vi "main.eng.proc-insert-instructions.vi"(8 "error in (no error)":errorcluster, 9 "instructions in":variant[](array[variant]), 10 "procedureName":string, 11 "procs in":cluster{"Procedure":variant[]}[](array[cluster])) -> (0 "error out":errorcluster, 3 "procs out":cluster{"Procedure":variant[]}[](array[cluster]))   [LabVIEW 2024]
uses:
  controls/typeProcVarientName.ctl
  Polymorphics/variantCtrlNumber.vi
  proc.util.validateParamExist.vi
  <vilib>/Utility/error.llb/Clear Errors.vi
  util.error.create.vi
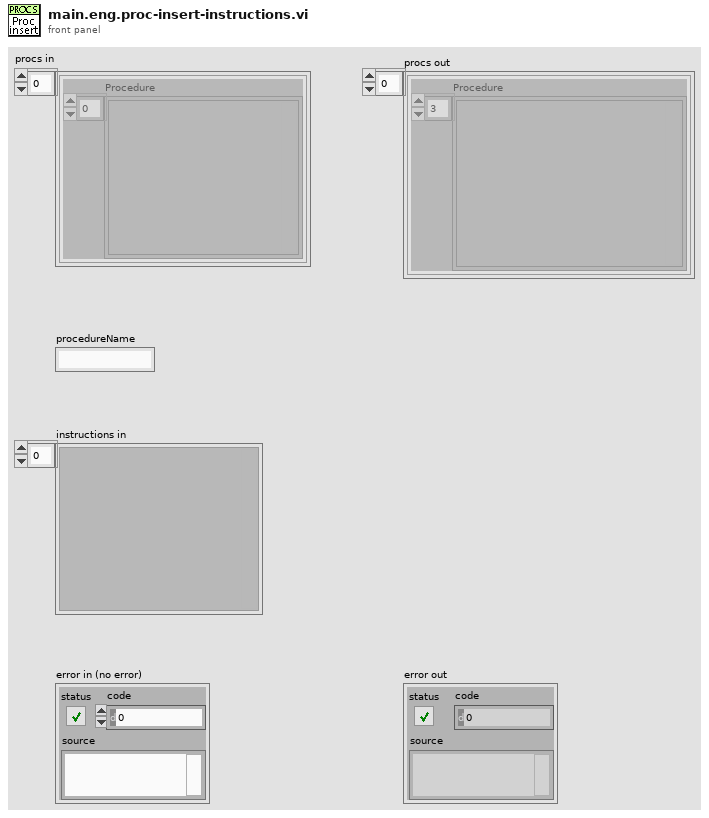
[diagram p1: front panel]
types:
  T1 = typedef "typeProcVarientName.ctl" = enum16{"procNameID", "procModuleID", "procPath", "procIsRunning", "procIndex", "procModule", "procRegisterNumeric", "procRegisterString", "procReport", "procReportPrev", "procCLK", "procStepPointer", "procType"}
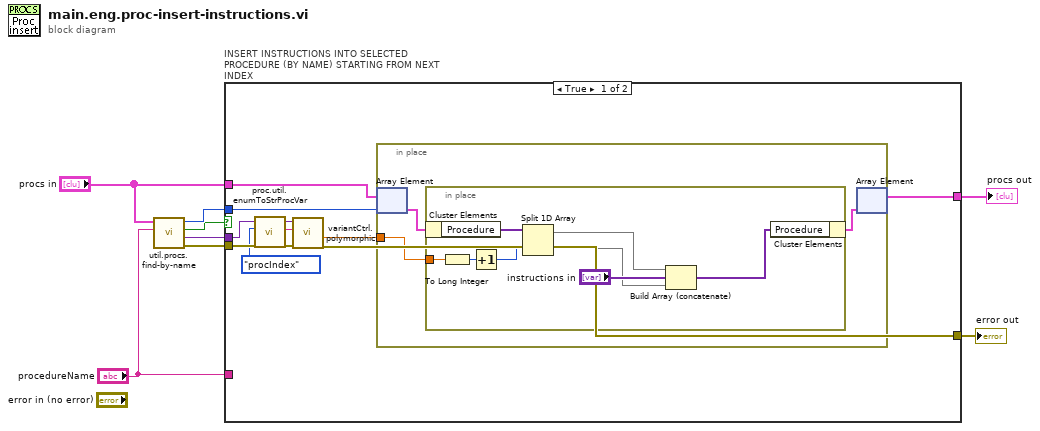
[diagram p0: block diagram]
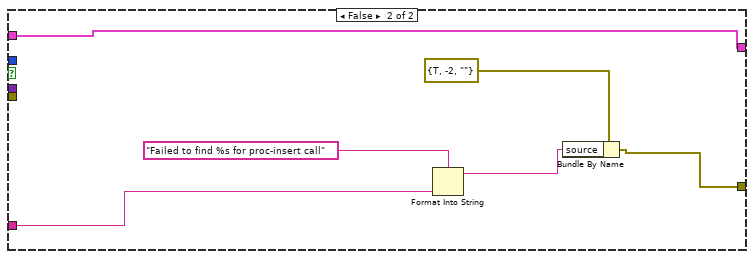
[diagram p2: hidden frame]
diagram:
  n1 = call "util.procs.find-by-name.vi"("ProcName in"="procedureName", "Procs in"="procs in") -> ("error out"=w3:errorcluster, "ProcHead"=w2:variant, "Found?"=w1:bool, "procIndex"=w5:i32)  [unwired: 4 in, 2 out]
  n2 = case "INSERT INSTRUCTIONS INTO SELECTED PROCEDURE (BY NAME) STARTING FROM NEXT INDEX" shown="True" w1 {
    tunnel: [w17 w34] -> w8
    tunnel: "procedureName" -> [_ w33]
    tunnel: "procs in" -> [w16 w32]
    tunnel: w5 -> [w15 _]
    tunnel: [w14 w32] -> w4
    tunnel: w3 -> [w13 _]
    tunnel: w2 -> [w12 _]
    frame True {
      n3 = call "proc.util.enumToStrProcVar.vi"("Proc var"=typeProcVarientName."procIndex" ("name")) -> ("String"=w10:string)  [unwired: 10 in]
      n4 = call-poly "variantCtrl.polymorphic.vi"("error in"=w13, "name in"=w10, "variant in"=w12) -> ("error out"=w17:errorcluster, "number"=w11:dbl)  [unwired: 5 in, 2 out]
      n5 = in-place {
        in-place-border: w11 -> [w20]
        n6 = in-place-array #1(w16, w15) -> (w19:cluster{"Procedure":variant[]})
        n7 = in-place {
          in-place-border: w20 -> [w28]
          n8 = in-place-cluster #2(w19) -> ("Procedure"=w26:variant[])
          n9 = To Long Integer(number=w28) -> (32bit integer=w25:i32)
          n10 = Increment(x=w25) -> (x+1=w21:i32)
          n11 = Split 1D Array(array=w26, index=w21) -> (first subarray=w24:variant[], second subarray=w23:variant[])
          n12 = Build Array (concatenate)(w24, "instructions in", w23) -> (w22:variant[])
          n13 = in-place-cluster #2("Procedure"=w22) -> (w18:cluster{"Procedure":variant[]})
        }
        n14 = in-place-array #1(w18) -> (w14:cluster{"Procedure":variant[]}[])  [unwired: 1 out]
      }
    }
    frame False {
      n15 = Format Into String(format string="Failed to find %s for proc-insert call" ("source"), w33) -> (resulting string=w29:string)  [unwired: 2 in, 1 out]
      n16 = Bundle By Name(cluster=errorcluster {"status"=TRUE, "code"=-2, "source"=""} ("error out"), "source"=w29) -> (w34:errorcluster)
    }
  }
  "error out" <- w8
  "procs out" <- w4
